vi "StreamHoldOn.vi"(8 "error in (no error)":errorcluster, 10 "StreamHoldOn":bool, 11 "Camera Actor in":refnum<class "Camera Actor.lvclass">) -> (0 "error out":errorcluster, 3 "Camera Actor out":refnum<class "Camera Actor.lvclass">)   [LabVIEW 2014, in "Camera Actor.lvlib" / "Camera Actor.lvclass"]
uses:
  Camera Actor.lvclass
  <vilib>/Utility/error.llb/DialogType.ctl
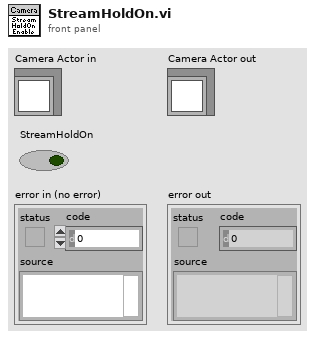
[diagram p1: front panel]
types:
  T1 = typedef "DialogType.ctl" = u16
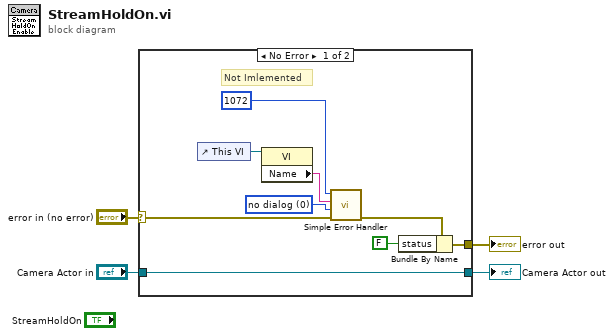
[diagram p0: block diagram]
diagram:
  n1 = case shown="No Error" "error in (no error)" {
    selector: "error in (no error)" -> [w12 w15]
    tunnel: [w8 w15] -> w3
    tunnel: [w13 w14] -> w1
    tunnel: "Camera Actor in" -> [w13 w14]
    frame No Error {
      w9 = T1 0 items=["no dialog", "OK message", "continue or stop message", "OK message + warnings", "continue/stop + warnings"] ("type of dialog (OK msg:1)")
      # "Not Imlemented"
      n2 = control-ref of="This VI"() -> (w6:refnum<vi>)
      n3 = property class="VI"(reference=w6) -> ("Name"=w5:string)  [unwired: 1 in, 2 out]
      n4 = call <vilib>:"Simple Error Handler.vi"("error code (no error:0)"=1072, "error source (\" \")"=w5, "type of dialog (OK msg:1)"=w9, "error in (no error)"=w12) -> ("error out"=w11:errorcluster)  [unwired: 1 in, 4 out]
      n5 = Bundle By Name(cluster=w11, "status"=FALSE) -> (w8:errorcluster)
    }
    frame Error {
    }
  }
  "error out" <- w3
  "Camera Actor out" <- w1
